vi "swabian_make_counter.vi"(8 "error in (no error)":errorcluster, 11 "swabian_local_data_IN":T1={"events"={"update_status"=refnum, "update_chart"=refnum, "update_xy"=refnum, "send_channel_data"=refnum}, "stop_q"=refnum, "tagger_reference"=refnum, "connect_button"=refnum, "counter_reference"=refnum, "tagger_stream_reference"=refnum, "log_reference"=refnum, "current_log_offset"=0, "tt20_buffer_q"=refnum, "stream_to_file_button"=refnum, "num_records"=0, "connected?"=FALSE, "plots"=refnum, "histogram_bin_edges"=[], "histogrammer"=refnum, "plot_lifetimes"=refnum, "xy_graph"=refnum, "Reference\nChannel"=enum."ch0", "trigger_channels"=[], "filter_channels"=[], "active_channels"=[], "acq_mode"=0, "Reference\nChannel"=enum."ch0", "acq_time"=0, "leftovers"={"leftover_stamps"=[], "leftover_channels"=[], "any?"=FALSE}, "sync_period_ps"=0, "raw_stream_path"=path "", "Leftovers"={"missing_sync_data"=[], "missing_events"=0}, "first_batch"=0, "first_sync_stamp"=0, "lifetime_settings"={"Plot Lifetimes"=FALSE, "start_time"=0.0, "stop_time"=0.0, "n_bins"=0}, "Histogram_bins"=[], "last_processed_data"=[], "histogram_data"=[]}) -> (0 "error out":errorcluster, 3 "swabian_local_data":T1={"events"={"update_status"=refnum, "update_chart"=refnum, "update_xy"=refnum, "send_channel_data"=refnum}, "stop_q"=refnum, "tagger_reference"=refnum, "connect_button"=refnum, "counter_reference"=refnum, "tagger_stream_reference"=refnum, "log_reference"=refnum, "current_log_offset"=0, "tt20_buffer_q"=refnum, "stream_to_file_button"=refnum, "num_records"=0, "connected?"=FALSE, "plots"=refnum, "histogram_bin_edges"=[], "histogrammer"=refnum, "plot_lifetimes"=refnum, "xy_graph"=refnum, "Reference\nChannel"=enum."ch0", "trigger_channels"=[], "filter_channels"=[], "active_channels"=[], "acq_mode"=0, "Reference\nChannel"=enum."ch0", "acq_time"=0, "leftovers"={"leftover_stamps"=[], "leftover_channels"=[], "any?"=FALSE}, "sync_period_ps"=0, "raw_stream_path"=path "", "Leftovers"={"missing_sync_data"=[], "missing_events"=0}, "first_batch"=0, "first_sync_stamp"=0, "lifetime_settings"={"Plot Lifetimes"=FALSE, "start_time"=0.0, "stop_time"=0.0, "n_bins"=0}, "Histogram_bins"=[], "last_processed_data"=[], "histogram_data"=[]})   [LabVIEW 2018]
uses:
  swabian_local_data_tdef.ctl
  swabian_events_tdef.ctl
  update_chart_tdef.ctl
  channel_data_tdef.ctl
  C:/Users/bspoka/Documents/swabian_LV/lib/TTCSharp32.dll
  lib/TTCSharp32.dll
  swabian_buffer_tdef.ctl
  reference_checkbox_tdef.ctl
  leftovers_struct.ctl
  lifetime_settings.ctl
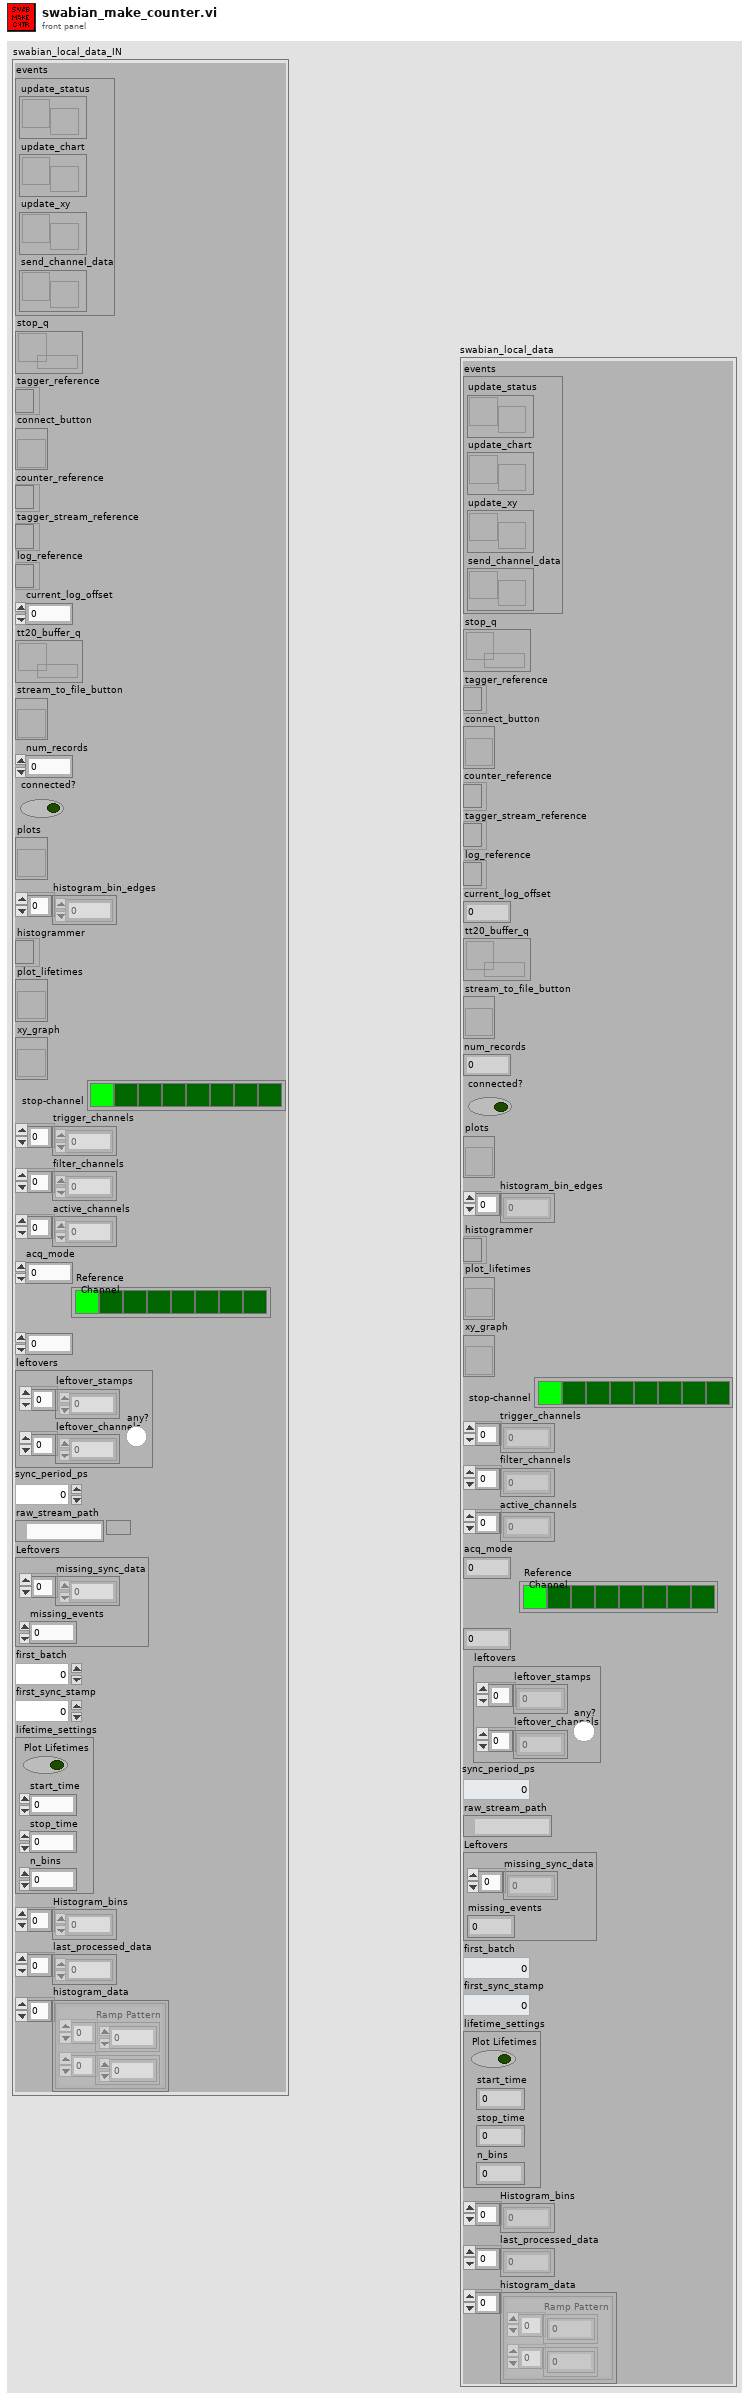
[diagram p1: front panel]
types:
  T1 = typedef "swabian_local_data_tdef.ctl" = cluster{"events":T2, "stop_q":refnum<queue>, "tagger_reference":refnum<k24>, "connect_button":refnum<vi>, "counter_reference":refnum<k24>, "tagger_stream_reference":refnum<k24>, "log_reference":refnum<file>, "current_log_offset":i64, "tt20_buffer_q":refnum<queue>, "stream_to_file_button":refnum<vi>, "num_records":u64, "connected?":bool, "plots":refnum<vi>, "histogram_bin_edges":i64[], "histogrammer":refnum<k24>, "plot_lifetimes":refnum<vi>, "xy_graph":refnum<vi>, "Reference\nChannel":T3, "trigger_channels":i32[], "filter_channels":i32[], "active_channels":i32[], "acq_mode":i32, "Reference\nChannel":T3, "acq_time":i64, "leftovers":T4, "sync_period_ps":i64, "raw_stream_path":path, "Leftovers":cluster{"missing_sync_data":u64[], "missing_events":i32}, "first_batch":i32, "first_sync_stamp":u64, "lifetime_settings":T5, "Histogram_bins":dbl[], "last_processed_data":u64[], "histogram_data":cluster{"Ramp Pattern":dbl[], dbl[]}[]}
  T2 = typedef "swabian_events_tdef.ctl" = cluster{"update_status":refnum<user-event>, "update_chart":refnum<user-event>, "update_xy":refnum<user-event>, "send_channel_data":refnum<user-event>}
  T3 = typedef "reference_checkbox_tdef.ctl" = enum32{"No Selection", "ch0", "ch1", "ch2", "ch3", "ch4", "ch5", "ch6", "ch7"}
  T4 = typedef "leftovers_struct.ctl" = cluster{"leftover_stamps":i64[], "leftover_channels":i32[], "any?":bool}
  T5 = typedef "lifetime_settings.ctl" = cluster{"Plot Lifetimes":bool, "start_time":dbl, "stop_time":dbl, "n_bins":i32}
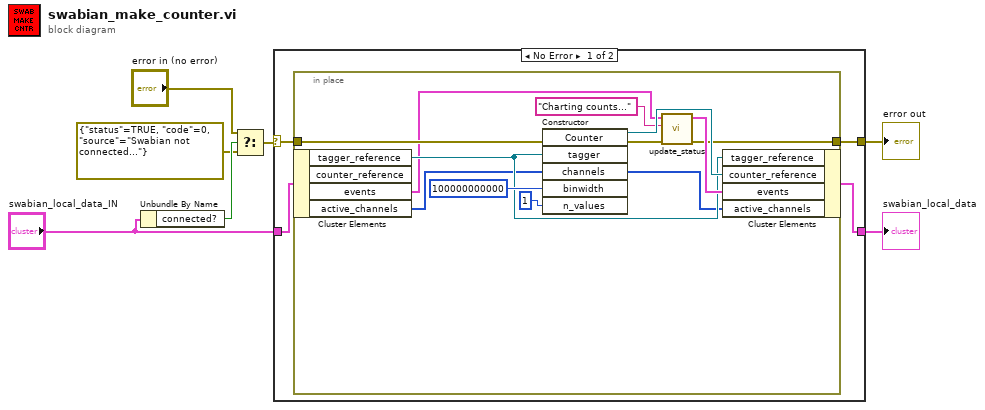
[diagram p0: block diagram]
diagram:
  n1 = Unbundle By Name("swabian_local_data_IN") -> ("connected?"=w5:bool)
  n2 = Select(t="error in (no error)", s=w5, f=errorcluster {"status"=TRUE, "code"=0, "source"="Swabian not connected..."}) -> (s? t:f=w1:errorcluster)
  n3 = case shown="No Error" w1 {
    selector: w1 -> [w10 w25]
    tunnel: "swabian_local_data_IN" -> [w11 w24]
    tunnel: [w9 w25] -> w7
    tunnel: [w8 w24] -> w6
    frame No Error {
      n4 = in-place {
        in-place-border: w10 -> [w19]
        in-place-border: [w17] -> w9
        n5 = in-place-cluster #1(w11) -> ("tagger_reference"=w18:refnum<k24>, "events"=w15:T2, "active_channels"=w13:i32[])  [unwired: 1 out]
        n6 = constructor class="Counter"(error in=w19, "tagger"=w18, "channels"=w13, "binwidth"=i64 100000000000, "n_values"=1) -> (reference out=w21:refnum<k24>, error out=w16:errorcluster, "channels"=w12:i32[])  [unwired: 2 in, 4 out]
        n7 = call "update_status.vi"("error in (no error)"=w16, "status"="Charting counts...", "events"=w15) -> ("error out"=w17:errorcluster, "events_out"=w23:T2)  [unwired: 7 in]
        n8 = in-place-cluster #1("tagger_reference"=w18, "counter_reference"=w21, "events"=w23, "active_channels"=w12) -> (w8:T1)
      }
    }
    frame Error {
    }
  }
  "error out" <- w7
  "swabian_local_data" <- w6
